vi "Scaffold INI Folder.vi"(8 "error in (no error)":errorcluster) -> (0 "error out":errorcluster, 3 "Scaffold INI Folder":path)   [LabVIEW 2020, in "Negentropic IDE.lvlib"]
uses:
  Negentropic IDE.lvlib
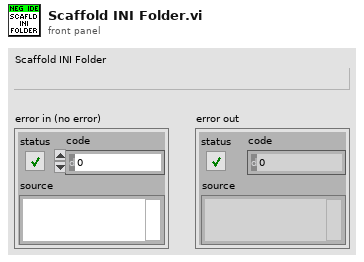
[diagram p1: front panel]
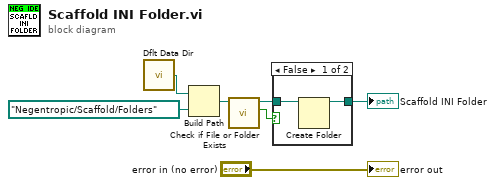
[diagram p0: block diagram]
diagram:
  n1 = call <vilib>:"Dflt Data Dir.vi"() -> ("App:Default Data Directory"=w7:path)
  n2 = Build Path(base path=w7, name or relative path=path "Negentropic/Scaffold/Folders") -> (appended path=w5:path)
  n3 = call <vilib>:"Check if File or Folder Exists.vi"("path"=w5) -> ("file or folder exists?"=w4:bool, "dup path"=w3:path)  [unwired: 8 in, 1 out]
  n4 = case shown="False" w4 {
    tunnel: w3 -> [w9 w10]
    tunnel: [w8 w10] -> w1
    frame False {
      n5 = Create Folder(path (use dialog)=w9) -> (created path=w8:path)  [unwired: 2 in, 2 out]
    }
    frame True {
    }
  }
  "Scaffold INI Folder" <- w1
  "error out" <- "error in (no error)"
